vi "Driver.vi"(7 "Square Inputs":bool, 11 "JoystickDevRef in":T1) -> (3 "JoystickDevRef out":T1)   [LabVIEW 2016]
uses:
  <vilib>/Rock Robotics/WPI/Joystick/WPI_JoystickDevRef.ctl
  <vilib>/Rock Robotics/WPI/Joystick/WPI_JoystickDeviceEnum.ctl
  <vilib>/Rock Robotics/Network Tables/NT Write Numeric Array.vi
  <vilib>/Rock Robotics/Network Tables/NT Write Boolean Array.vi
  Robot Values.vi
  LED Send Global.vi
panel:
  in  "Drive Divider":dbl=0.5
  # "Joysticks"
  # "Motor output"
  # "Inputs"
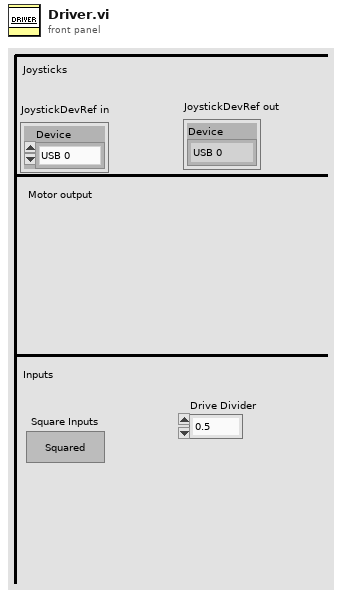
[diagram p1: front panel]
types:
  T1 = typedef "WPI_JoystickDevRef.ctl" = cluster{"Device":T2}
  T2 = typedef "WPI_JoystickDeviceEnum.ctl" = enum16{"USB 0", "USB 1", "USB 2", "USB 3", "USB 4", "USB 5"}
  T3 = typedef "Robot Values.ctl" = cluster{"Robot Drive":cluster{"Left Motor Power":dbl, "Right Motor Power":dbl, "Left Encoder Value":dbl, "Right Encoder Value":dbl, "High Gear?":bool, "PTO?":bool}, "Sensors":cluster{"Gyro Angle":u16, "Recalibrate Gyro":bool, "Reset Gyro":bool, "Ultrasonic":dbl}, "Shooter":cluster{"Prep Wheels":bool, "Shoot":bool, "Left Shooter Wheel Speed":dbl, "Wheels Moving":bool, "Shooter Prepped":bool, "Shooter RPS SP":dbl, "Shooting?":bool, "Left Shooter Wheel Power":dbl, "Right Shooter Wheel Power":dbl, "Acquisition Conveyor Power":dbl, "Hopper Beater Bar Power":dbl, "Filtered Left Shooter Speed":dbl, "Acquisition Motor Power":dbl, "Joystick Add":dbl, "D-Pad Add":dbl, "Shooter Use PID?":bool}, "Robot States":cluster{"Drive mode":string, "Alliance":T4, "Position":T5}, "Gear":cluster{"Ejection Active":bool}}
  T4 = typedef "WPI_DriverStationAllianceInfo.ctl" = enum16{"Red", "Blue", "Invalid"}
  T5 = typedef "WPI_DriverStationPositionInfo.ctl" = enum16{"1", "2", "3"}
  T6 = cluster{"Start  Button":bool, "Back Button":bool, "Left Trigger":bool, "Left  Bumper":bool, "Right Trigger":bool, "Right Bumper":bool, "A Button":bool, "B Button":bool, "X Button":bool, "Y Button":bool, "Left Joystick Press":bool, "Right Joystick Press":bool}
  T7 = typedef "LED Send Global.ctl" = cluster{"Underglow States":cluster{"RED":bool, "BLUE":bool}, "Hopper States":cluster{"No Shooter Power":bool, "1 RED":bool, "2 RED":bool, "3 RED":bool, "1 YEL 3 RED":bool, "2 YEL 3 RED":bool, "3 YEL 3 RED":bool, "1 GRN 3 YEL 3 RED":bool, "2 GRN 3 YEL 3 RED":bool, "3 GRN 3 YEL 3 RED":bool, "All GRN":bool, "Shooter w/Agitator":bool}, "License Plate States":cluster{"Auton States":cluster{"Do Nothing":bool, "Gear":bool, "Gear & Baseline":bool, "Gear & Shooter":bool, "Shooter":bool, "Shooter & Ball Dump":bool}, "Drive Train":cluster{"High Gear":bool, "Low Gear":bool}}, "Misc":cluster{"Pit/Demo":bool}, "Lights":cluster{"Underglow":string, "License Plate":string, "Hopper":string}}
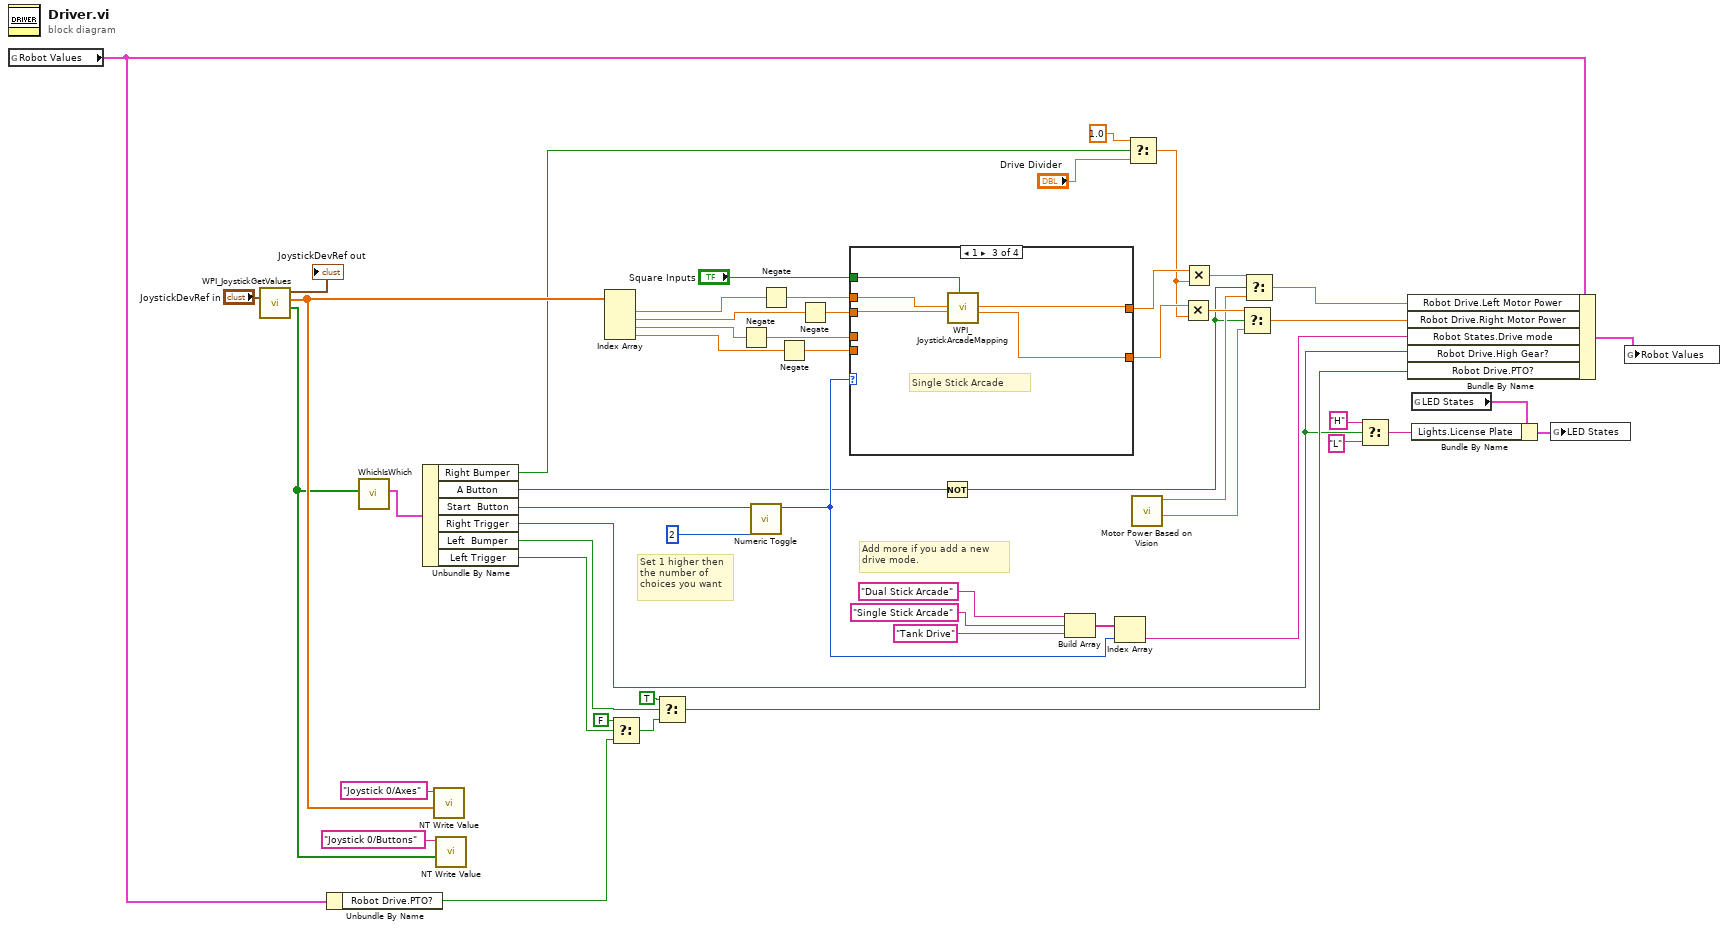
[diagram p0: block diagram]
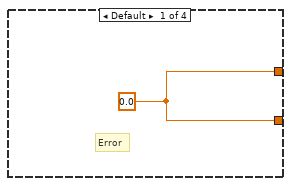
[diagram p2: hidden frame]
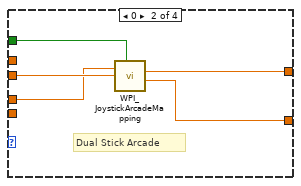
[diagram p3: hidden frame]
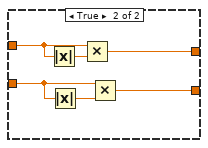
[diagram p5: hidden frame]
diagram:
  # "Add more if you add a new \ndrive mode."
  # "Set 1 higher then \nthe number of \nchoices you want"
  n1 = global read "Robot Values.vi" "Robot Values"() -> (w22:T3)
  n2 = call <vilib>:"WPI_JoystickGetValues.vi"("JoystickDevRef"="JoystickDevRef in") -> ("Buttons"=w35:bool[], "Axes"=w51:dbl[], "JoystickDevRef"=→"JoystickDevRef out":T1)  [unwired: 6 in, 2 out]
  n3 = Unbundle By Name(w22) -> ("Robot Drive.PTO?"=w21:bool)
  n4 = call "WhichIsWhich.vi"("Button Values Array"=w35) -> ("Button Values Cluster"=w34:T6)  [unwired: 8 in]
  n5 = Unbundle By Name(w34) -> ("Right Bumper"=w17:bool, "A Button"=w8:bool, "Start  Button"=w33:bool, "Right Trigger"=w14:bool, "Left  Bumper"=w32:bool, "Left Trigger"=w28:bool)
  n6 = call-poly <vilib>:"NT Write Value.vi"("Numeric Array"=w51, "Name"="Joystick 0/Axes") -> ()  [unwired: 9 in, 1 out]
  n7 = call-poly <vilib>:"NT Write Value.vi"("Boolean Array"=w35, "Name"="Joystick 0/Buttons") -> ()  [unwired: 9 in, 1 out]
  n8 = Index Array(array=w51) -> (element #1=w49:dbl, element #2=w48:dbl, element #3=w47:dbl, element #4=w46:dbl)  [unwired: 4 in]
  n9 = Select(t=FALSE, s=w28, f=w21) -> (s? t:f=w30:bool)
  n10 = Select(t=TRUE, s=w32, f=w30) -> (s? t:f=w27:bool)
  n11 = Negate(x=w47) -> (-x=w24:dbl)
  n12 = call "Numeric Toggle.vi"("# of Cases"=2, "Toggle Input"=w33) -> ("Output"=w44:i32)  [unwired: 9 in]
  n13 = Negate(x=w49) -> (-x=w26:dbl)
  n14 = Negate(x=w46) -> (-x=w23:dbl)
  n15 = Negate(x=w48) -> (-x=w25:dbl)
  n16 = case shown="1" w44 {
    tunnel: w26 -> [_ _ w64 _]
    tunnel: w25 -> [_ w59 w63 w68]
    tunnel: [w54 w58 w62 w66] -> w20
    tunnel: [w54 w57 w61 w65] -> w19
    tunnel: w24 -> [_ w56 _ _]
    tunnel: w23 -> [_ _ _ w67]
    tunnel: "Square Inputs" -> [_ w55 w60 w69]
    frame Default {
      w54 = 0.0 ("Left Motor Value")
      # "Error"
    }
    frame 0 {
      # "Dual Stick Arcade"
      n17 = call <vilib>:"WPI_JoystickArcadeMapping.vi"("Square Inputs"=w55, "Y axis value"=w59, "X axis value"=w56) -> ("Right Motor Value"=w57:dbl, "Left Motor Value"=w58:dbl)  [unwired: 7 in]
    }
    frame 1 {
      # "Single Stick Arcade"
      n18 = call <vilib>:"WPI_JoystickArcadeMapping.vi"("Square Inputs"=w60, "Y axis value"=w63, "X axis value"=w64) -> ("Right Motor Value"=w61:dbl, "Left Motor Value"=w62:dbl)  [unwired: 7 in]
    }
    frame 2 {
      # "Tank Drive"
      n19 = case shown="False" w69 {
        tunnel: w68 -> [w71 w76]
        tunnel: w67 -> [w70 w75]
        tunnel: [w71 w77] -> w66
        tunnel: [w70 w74] -> w65
        frame False {
        }
        frame True {
          n20 = Absolute Value(x=w76) -> (abs(x)=w73:dbl)
          n21 = Absolute Value(x=w75) -> (abs(x)=w72:dbl)
          n22 = Multiply(x=w76, y=w73) -> (x*y=w77:dbl)
          n23 = Multiply(x=w75, y=w72) -> (x*y=w74:dbl)
        }
      }
    }
  }
  n24 = Not(x=w8) -> (.not. x?=w1:bool)
  n25 = Build Array("Dual Stick Arcade", "Single Stick Arcade", "Tank Drive") -> (w43:string[])
  n26 = Index Array(array=w43, index=w44) -> (element=w36:string)
  n27 = Select(t=1.0 ("f"), s=w17, f="Drive Divider") -> (s? t:f=w18:dbl)
  n28 = call "Motor Power Based on Vision.vi"() -> ("Right Motor Power"=w2:dbl, "Left Motor Power"=w3:dbl)  [unwired: 10 in]
  n29 = Multiply(x=w19, y=w18) -> (x*y=w5:dbl)
  n30 = Multiply(x=w20, y=w18) -> (x*y=w7:dbl)
  n31 = Select(t=w5, s=w1, f=w2) -> (s? t:f=w4:dbl)
  n32 = Select(t=w7, s=w1, f=w3) -> (s? t:f=w6:dbl)
  n33 = Select(t="H", s=w14, f="L") -> (s? t:f=w11:string)
  n34 = Bundle By Name(cluster=w22, "Robot Drive.Left Motor Power"=w6, "Robot Drive.Right Motor Power"=w4, "Robot States.Drive mode"=w36, "Robot Drive.High Gear?"=w14, "Robot Drive.PTO?"=w27) -> (w37:T3)
  n35 = global read "LED Send Global.vi" "LED States"() -> (w12:T7)
  n36 = Bundle By Name(cluster=w12, "Lights.License Plate"=w11) -> (w13:T7)
  n37 = global write "LED Send Global.vi" "LED States"(w13) -> ()
  n38 = global write "Robot Values.vi" "Robot Values"(w37) -> ()
